vi "cmd_advanced_scan.vi"(8 "error in (no error)":errorcluster, 11 "JSON":string) -> (0 "error out":errorcluster)   [LabVIEW 2021]
doc: "Call advanced_scan command\n\n Before use this command, we need to move the analog outputs to an inital position.\n When you want to use auto_reversal mode, please also call set_threshold command before this command.\n\n :param nx: Specifies the number of fast scan points\n :param ny: Specifies the number of slow scan points\n :param dx: Specifies the delta for fast scan (8ch)\n :param dy: Specifies the delta for slow scan (8ch)\n :param avg: Specifies the average counts\n :param bidirectional: Bidirectional scan flag\n :param auto_reversal: Auto reversal flag\n :return: None"
uses:
  fpga/fpga_dtype_scan_config.ctl
  fpga/fpga_dtype_sgl_8ch.ctl
  fpga/fpga_dtype_index.ctl
panel:
  in  "args":T1
  # "Before call this function,\nplease move analog output to an initial position."
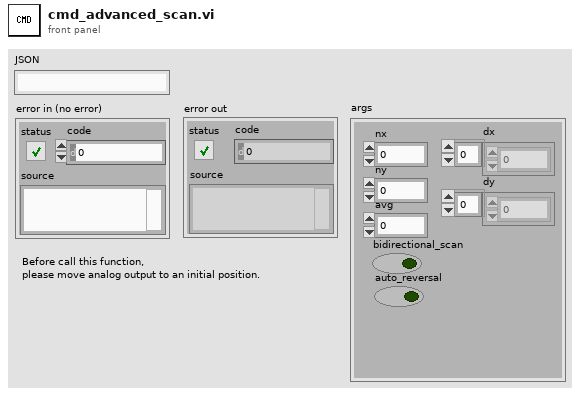
[diagram p1: front panel]
types:
  T1 = cluster{"nx":i32, "ny":i32, "avg":i32, "bidirectional_scan":bool, "auto_reversal":bool, "dx":sgl[], "dy":sgl[]}
  T2 = typedef "fpga_dtype_index.ctl" = cluster{"page":i16, "2nd":i16, "1st":i16}
  T3 = typedef "fpga_dtype_scan_config.ctl" = cluster{"data points":i16, "average counts":i16, "delta per point":T4, "bidirectional scan":bool, "auto reversal":bool}
  T4 = typedef "fpga_dtype_sgl_8ch.ctl" = cluster{"ch 0":sgl, "ch 1":sgl, "ch 2":sgl, "ch 3":sgl, "ch 4":sgl, "ch 5":sgl, "ch 6":sgl, "ch 7":sgl}
  T5 = cluster{"dx[0]":sgl, "dx[1]":sgl, "dx[2]":sgl, "dx[3]":sgl, "dx[4]":sgl, "dx[5]":sgl, "dx[6]":sgl, "dx[7]":sgl}
  T6 = cluster{"[0]":sgl, "[1]":sgl, "[2]":sgl, "[3]":sgl, "[4]":sgl, "[5]":sgl, "[6]":sgl, "[7]":sgl}
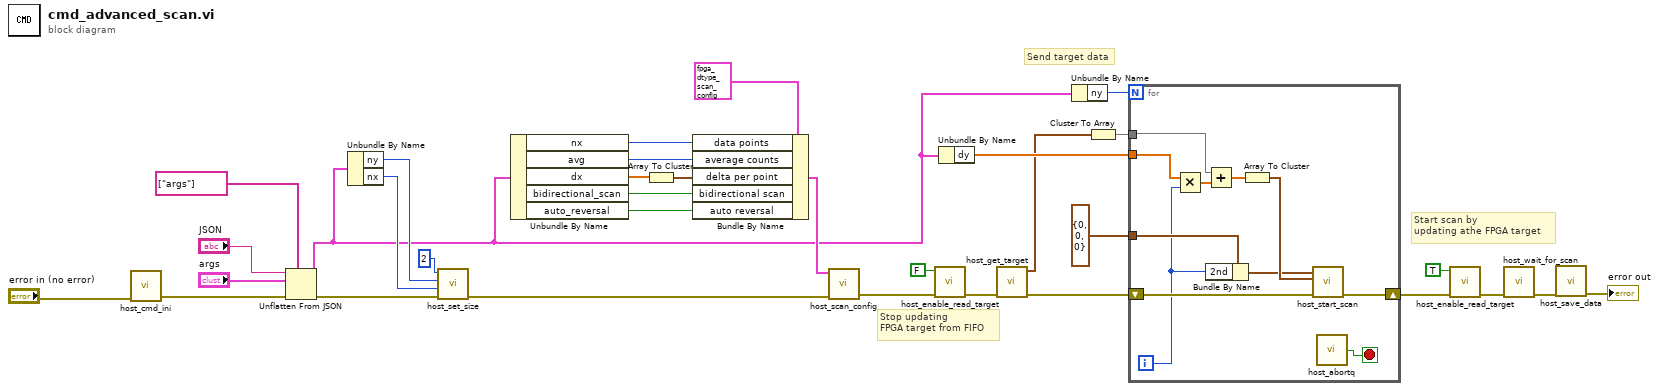
[diagram p0: block diagram]
diagram:
  # "Start scan by\nupdating athe FPGA target"
  # "Send target data"
  # "Stop updating \nFPGA target from FIFO"
  n1 = call "host_cmd_ini.vi"("error in (no error)"="error in (no error)") -> ("error out"=w18:errorcluster)  [unwired: 10 in]
  n2 = Unflatten From JSON(path=string[] ["args"], JSON string="JSON", type and defaults="args", error in (no error)=w18) -> (value=w11:T1, error out=w27:errorcluster)  [unwired: 3 in]
  n3 = Unbundle By Name(w11) -> ("ny"=w24:i32, "nx"=w23:i32)
  n4 = call "host_set_size.vi"("error in (no error)"=w27, "fast"=w23, "slow"=w24, "page"=2) -> ("error out"=w26:errorcluster)  [unwired: 7 in]
  n5 = Unbundle By Name(w11) -> ("nx"=w20:i32, "avg"=w28:i32, "dx"=w14:sgl[], "bidirectional_scan"=w16:bool, "auto_reversal"=w15:bool)
  n6 = Array To Cluster(array=w14) -> (cluster=w13:T5)
  n7 = Bundle By Name(cluster=T3 {"data points"=0, "average counts"=0, "delta per point"={"ch 0"=0.0, "ch 1"=0.0, "ch 2"=0.0, "ch 3"=0.0, "ch 4"=0.0, "ch 5"=0.0, "ch 6"=0.0, "ch 7"=0.0}, "bidirectional scan"=FALSE, "auto reversal"=FALSE} ("scan config"), "data points"=w20, "average counts"=w28, "delta per point"=w13, "bidirectional scan"=w16, "auto reversal"=w15) -> (w12:T3)
  n8 = call "host_scan_config.vi"("error in"=w26, "scan config"=w12) -> ("error out"=w5:errorcluster)  [unwired: 9 in]
  n9 = call "host_enable_read_target.vi"("error in"=w5, "enable read target?"=FALSE) -> ("error out"=w6:errorcluster)  [unwired: 9 in]
  n10 = Unbundle By Name(w11) -> ("dy"=w10:sgl[])
  n11 = call "host_get_target.vi"("error in"=w6) -> ("error out"=w21:errorcluster, "target"=w9:T4)  [unwired: 9 in]
  n12 = Unbundle By Name(w11) -> ("ny"=w22:i32)
  n13 = Cluster To Array(cluster=w9) -> (array=w8:sgl[])
  n14 = for {
    N: w22 -> [_]
    shift-right: [w42] -> w3
    shift-left: w21 -> [w43]
    tunnel: w10 -> [w40]
    tunnel: w8 -> [w39]
    tunnel: T2 {"page"=0, "2nd"=0, "1st"=0} ("index offset") -> [w36]
    i -> [w34]
    stop <- w44 stop-if-true
    n15 = Multiply(x=w40, y=w34) -> (x*y=w41:sgl[])
    n16 = Add(x=w39, y=w41) -> (x+y=w38:sgl[])
    n17 = Bundle By Name(cluster=w36, "2nd"=w34) -> (w35:T2)
    n18 = Array To Cluster(array=w38) -> (cluster=w37:T6)
    n19 = call "host_start_scan.vi"("error in"=w43, "initial positions"=w37, "index offset"=w35) -> ("error out"=w42:errorcluster)  [unwired: 6 in, 2 out]
    n20 = call "host_abortq.vi"() -> ("abort"=w44:bool)  [unwired: 1 in]
  }
  n21 = call "host_enable_read_target.vi"("error in"=w3, "enable read target?"=TRUE) -> ("error out"=w2:errorcluster)  [unwired: 9 in]
  n22 = call "host_wait_for_scan.vi"("error in (no error)"=w2) -> ("error out"=w19:errorcluster)  [unwired: 10 in]
  n23 = call "host_save_data.vi"("error in"=w19) -> ("error out"=→"error out":errorcluster)  [unwired: 10 in]
